vi "Scale Data.vi"(8 "error in (no error)":errorcluster, 9 "Scaling Info":T1, 10 "Raw Value":u64 format="%064b") -> (0 "error out":errorcluster, 2 "Scaled Value":dbl)   [LabVIEW 2020, in "BCI-1553 API.lvlib"]
doc: "Converts from a raw U64 representation of a value to a double. The actual final scaled value will depend entirely on the the contents of the Scaling Info cluster."
uses:
  BCI-1553 API.lvlib
  TypeDefs/Scaling Information.ctl
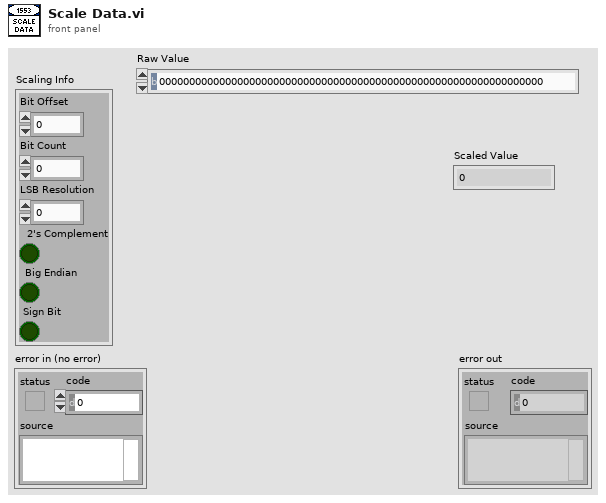
[diagram p1: front panel]
types:
  T1 = typedef "BCI-1553 API.lvlib/Scaling Information.ctl" = cluster{"Bit Offset":i32, "Bit Count":i32, "LSB Resolution":dbl, "2's Complement":bool, "Big Endian":bool, "Sign Bit":bool}
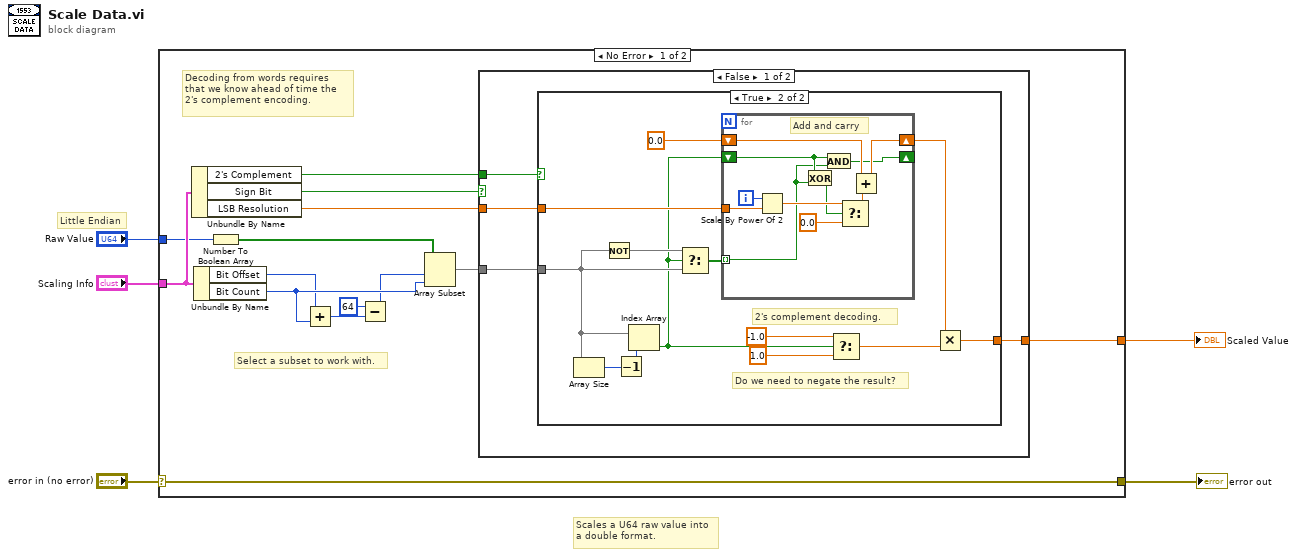
[diagram p0: block diagram]
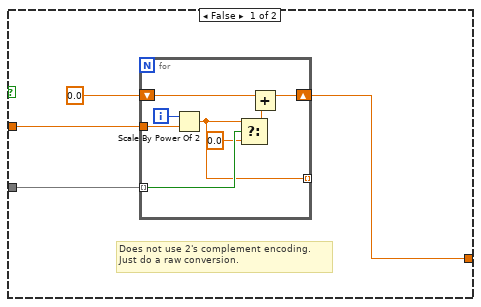
[diagram p2: hidden frame]
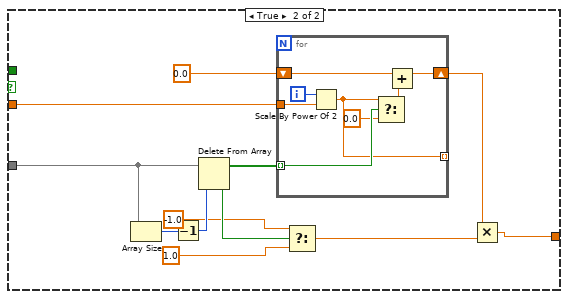
[diagram p3: hidden frame]
diagram:
  # "Little Endian"
  # "Scales a U64 raw value into\na double format."
  n1 = case shown="No Error" "error in (no error)" {
    selector: "error in (no error)" -> [w19 w80]
    tunnel: [w19 w80] -> w4
    tunnel: "Raw Value" -> [w15 _]
    tunnel: "Scaling Info" -> [w18 _]
    tunnel: [w16 _] -> w1
    frame No Error {
      # "Decoding from words requires\nthat we know ahead of time the\n2's complement encoding."
      # "Select a subset to work with."
      n2 = Unbundle By Name(w18) -> ("2's Complement"=w7:bool, "Sign Bit"=w6:bool, "LSB Resolution"=w17:dbl)
      n3 = Unbundle By Name(w18) -> ("Bit Offset"=w9:i32, "Bit Count"=w10:i32)
      n4 = Number To Boolean Array(number=w15) -> (Boolean array=w14:bool[])
      n5 = Add(x=w9, y=w10) -> (x+y=w11:i32)
      n6 = Subtract(x=64 ("dimension size"), y=w11) -> (x-y=w8:i32)
      n7 = Array Subset(array=w14, index=w8, length=w10) -> (w13:bool[])
      n8 = case shown="False" w6 {
        tunnel: w17 -> [w23 w62]
        tunnel: w13 -> [w21 w61]
        tunnel: [w22 w60] -> w16
        tunnel: w7 -> [w20 _]
        frame False {
          n9 = case shown="True" w20 {
            tunnel: w23 -> [w26 w46]
            tunnel: [w24 w44] -> w22
            tunnel: w21 -> [w25 w38]
            frame False {
              # "Does not use 2's complement encoding.\nJust do a raw conversion."
              n10 = for {
                tunnel: w25 -> [w32] mode=indexing
                tunnel: w26 -> [w34]
                shift-right: [w29] -> w24
                shift-left: 0.0 -> [w30]
                tunnel: [w28] -> _ mode=indexing
                i -> [w35]
                n11 = Scale By Power Of 2(n=w35, x=w34) -> (x*2^n=w28:dbl)
                n12 = Select(t=w28, s=w32, f=0.0) -> (s? t:f=w33:dbl)
                n13 = Add(x=w30, y=w33) -> (x+y=w29:dbl)
              }
            }
            frame True {
              # "Do we need to negate the result?"
              # "2's complement decoding."
              n14 = Array Size(array=w38) -> (size(s)=w41:i32)
              n15 = Not(x=w38) -> (.not. x?=w39:bool[])
              n16 = Decrement(x=w41) -> (x-1=w40:i32)
              n17 = Index Array(array=w38, index=w40) -> (element=w36:bool)
              n18 = Select(t=w39, s=w36, f=w38) -> (s? t:f=w37:bool[])
              n19 = for {
                tunnel: w37 -> [w49] mode=indexing
                tunnel: w46 -> [w58]
                shift-right: [w51] -> w43
                shift-left: 0.0 -> [w54]
                shift-right: [w50] -> _
                shift-left: w36 -> [w57]
                i -> [w59]
                # "Add and carry"
                n20 = Scale By Power Of 2(n=w59, x=w58) -> (x*2^n=w55:dbl)
                n21 = Exclusive Or(1:w49, 2:w57) -> (0:w53:bool)
                n22 = And(x=w57, y=w49) -> (x .and. y?=w50:bool)
                n23 = Select(t=w55, s=w53, f=0.0) -> (s? t:f=w52:dbl)
                n24 = Add(x=w54, y=w52) -> (x+y=w51:dbl)
              }
              n25 = Select(t=-1.0, s=w36, f=1.0) -> (s? t:f=w45:dbl)
              n26 = Multiply(x=w43, y=w45) -> (x*y=w44:dbl)
            }
          }
        }
        frame True {
          n27 = Array Size(array=w61) -> (size(s)=w69:i32)
          n28 = Decrement(x=w69) -> (x-1=w68:i32)
          n29 = Delete From Array(array=w61, index=w68) -> (deleted portion=w67:bool, array with subset deleted=w70:bool[])  [unwired: 1 in]
          n30 = for {
            tunnel: w70 -> [w76] mode=indexing
            tunnel: w62 -> [w78]
            shift-right: [w73] -> w63
            shift-left: 0.0 -> [w74]
            tunnel: [w72] -> _ mode=indexing
            i -> [w79]
            n31 = Scale By Power Of 2(n=w79, x=w78) -> (x*2^n=w72:dbl)
            n32 = Select(t=w72, s=w76, f=0.0) -> (s? t:f=w77:dbl)
            n33 = Add(x=w74, y=w77) -> (x+y=w73:dbl)
          }
          n34 = Select(t=-1.0, s=w67, f=1.0) -> (s? t:f=w64:dbl)
          n35 = Multiply(x=w63, y=w64) -> (x*y=w60:dbl)
        }
      }
    }
    frame Error {
    }
  }
  "error out" <- w4
  "Scaled Value" <- w1
